vi "AuxSetCurrent.vi"(6 "Enabled?":bool=TRUE, 8 "error in":errorcluster, 9 "VISA resource name":refnum<visa-resource-name>="COM8", 10 "Function select":enum16{"Init", "Set", "Close"}(ring)=enum."Set", 11 "current /mA":dbl) -> (0 "error out":errorcluster, 1 "VISA resource name out":refnum<visa-resource-name>, 3 "output str":string)   [LabVIEW 2019]
uses:
  <vilib>/Instr/_visa.llb/VISA Configure Serial Port (Instr).vi
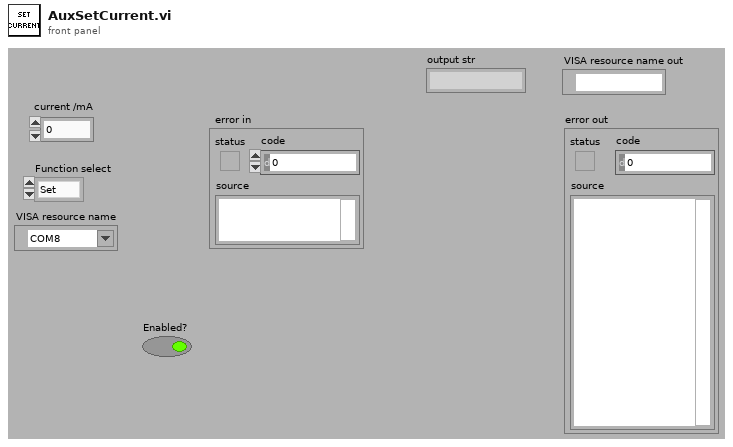
[diagram p1: front panel]
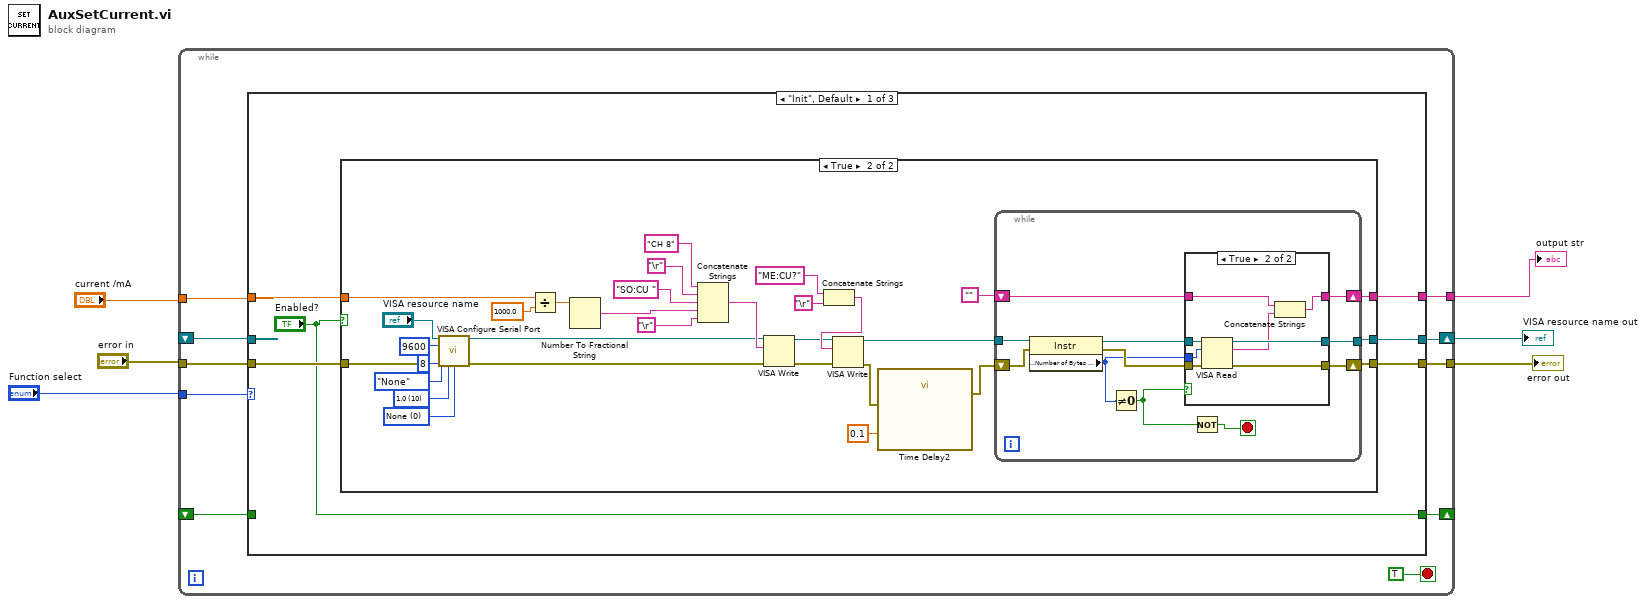
[diagram p0: block diagram]
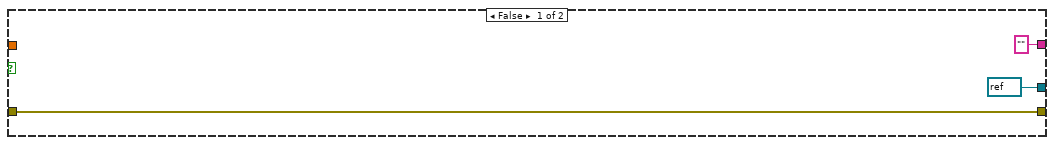
[diagram p2: hidden frame]
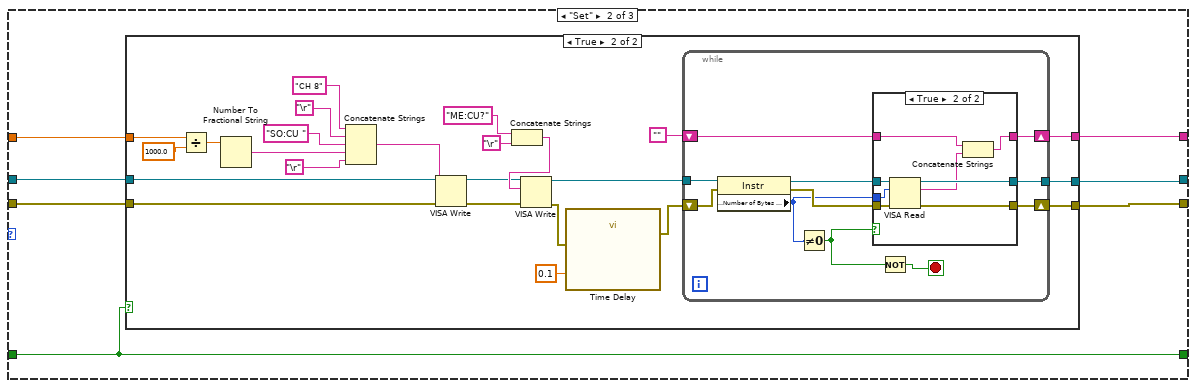
[diagram p4: hidden frame]
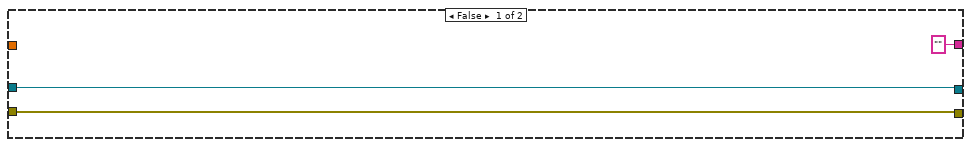
[diagram p5: hidden frame]
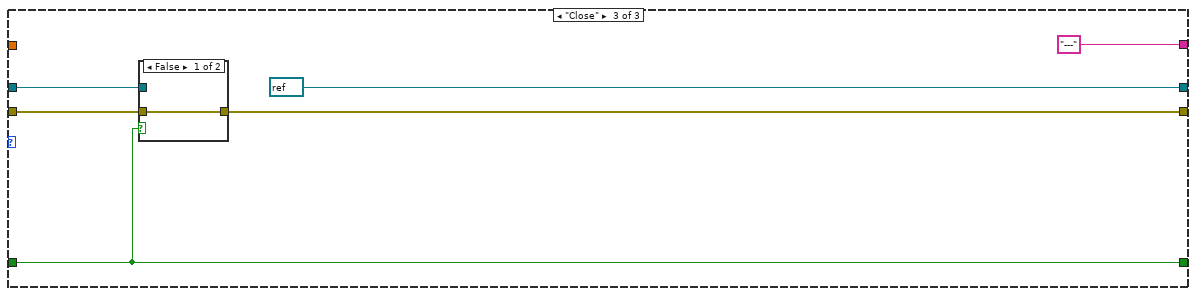
[diagram p7: hidden frame]
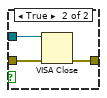
[diagram p8: hidden frame]
diagram:
  n1 = while {
    shift-right: [w15] -> w2
    shift-left: _ -> [w14]
    tunnel: "Function select" -> [w13]
    tunnel: "current /mA" -> [w12]
    tunnel: [w11] -> w4
    tunnel: "error in" -> [w10]
    tunnel: [w9] -> w1
    shift-right: [w8] -> _
    shift-left: _ -> [w7]
    stop <- TRUE stop-if-true
    n2 = case shown="\"Init\", Default" w13 {
      tunnel: [w19 w82 refnum<visa-resource-name> refnum ("VISA resource name out")] -> w15
      tunnel: w14 -> [_ w83 w140]
      tunnel: w12 -> [w21 w85 _]
      tunnel: [w18 w81 w137] -> w11
      tunnel: w10 -> [w22 w84 w138]
      tunnel: [w20 w80 "---"] -> w9
      tunnel: ["Enabled?" w79 w135] -> w8
      tunnel: w7 -> [_ w79 w135]
      frame "Init", Default {
        n3 = case shown="True" "Enabled?" {
          tunnel: w22 -> [w24 w50]
          tunnel: w21 -> [_ w39]
          tunnel: ["" w29] -> w20
          tunnel: [refnum<visa-resource-name> refnum ("VISA resource name out") w28] -> w19
          tunnel: [w24 w27] -> w18
          frame False {
          }
          frame True {
            w56 = u16 0 items=["None", "XON/XOFF", "RTS/CTS", "XON/XOFF & RTS/CTS", "DTR/DSR", "XON/XOFF & DTR/DSR"] ("flow control (0:none)")
            w55 = u16 10 items=["1.0"=10, "1.5"=15, "2.0"=20] ("stop bits (10: 1 bit)")
            n4 = call-poly "VISA Configure Serial Port"("VISA resource name"="VISA resource name", "baud rate (9600)"=u32 9600, "data bits (8)"=u16 8, "parity (0:none)"=enum16{"None", "Odd", "Even", "Mark", "Space"}."None", "error in (no error)"=w50, "stop bits (10: 1 bit)"=w55, "flow control (0:none)"=w56) -> ("VISA resource name out"=w40:refnum<visa-resource-name>, "error out"=w41:errorcluster)  [unwired: 7 in]
            n5 = Divide(x=w39, y=1000.0) -> (x/y=w45:dbl)
            n6 = Number To Fractional String(number=w45) -> (F-format string=w42:string)  [unwired: 3 in]
            n7 = Concatenate Strings("CH 8" ("write buffer"), "\r", "SO:CU ", w42, "\r") -> (w46:string)
            n8 = VISA Write(VISA resource name=w40, write buffer=w46, error in (no error)=w41) -> (VISA resource name out=w31:refnum<visa-resource-name>, error out=w30:errorcluster)  [unwired: 1 out]
            n9 = Concatenate Strings("ME:CU?" ("write buffer"), "\r") -> (w35:string)
            n10 = VISA Write(VISA resource name=w31, write buffer=w35, error in (no error)=w30) -> (VISA resource name out=w36:refnum<visa-resource-name>, error out=w38:errorcluster)  [unwired: 1 out]
            n11 = call "Time Delay2"("error in (no error)"=w38, "Delay Time (s)"=0.1) -> ("error out"=w37:errorcluster)  [unwired: 9 in]
            n12 = while {
              tunnel: w36 -> [w66]
              tunnel: [w63] -> w28
              shift-right: [w62] -> w27
              shift-left: w37 -> [w67]
              shift-right: [w57] -> w29
              shift-left: "" -> [w58]
              stop <- w60 stop-if-true
              n13 = property class="Instr"(reference=w66, error in=w67) -> (reference out=w65:refnum<visa-resource-name>, error out=w64:errorcluster, "Serial Settings:Number of Bytes at Serial Port"=w61:u32)
              n14 = Not Equal To 0?(x=w61) -> (x != 0?=w59:bool)
              n15 = case shown="True" w59 {
                tunnel: w65 -> [w70 w78]
                tunnel: w64 -> [w69 w77]
                tunnel: [w70 w75] -> w63
                tunnel: [w69 w74] -> w62
                tunnel: w61 -> [_ w76]
                tunnel: w58 -> [w68 w73]
                tunnel: [w68 w71] -> w57
                frame False {
                }
                frame True {
                  n16 = VISA Read(VISA resource name=w78, byte count=w76, error in (no error)=w77) -> (VISA resource name out=w75:refnum<visa-resource-name>, read buffer=w72:string, error out=w74:errorcluster)  [unwired: 1 out]
                  n17 = Concatenate Strings(w73, w72) -> (w71:string)
                }
              }
              n18 = Not(x=w59) -> (.not. x?=w60:bool)
            }
          }
        }
      }
      frame "Set" {
        n19 = case shown="True" w79 {
          tunnel: w85 -> [_ w104]
          tunnel: w84 -> [w88 w103]
          tunnel: w83 -> [w87 w102]
          tunnel: [w87 w91] -> w82
          tunnel: [w88 w90] -> w81
          tunnel: ["" w89] -> w80
          frame False {
          }
          frame True {
            n20 = Divide(x=w104, y=1000.0) -> (x/y=w108:dbl)
            n21 = Number To Fractional String(number=w108) -> (F-format string=w105:string)  [unwired: 3 in]
            n22 = Concatenate Strings("CH 8" ("write buffer"), "\r", "SO:CU ", w105, "\r") -> (w109:string)
            n23 = VISA Write(VISA resource name=w102, write buffer=w109, error in (no error)=w103) -> (VISA resource name out=w93:refnum<visa-resource-name>, error out=w92:errorcluster)  [unwired: 1 out]
            n24 = Concatenate Strings("ME:CU?" ("write buffer"), "\r") -> (w98:string)
            n25 = VISA Write(VISA resource name=w93, write buffer=w98, error in (no error)=w92) -> (VISA resource name out=w96:refnum<visa-resource-name>, error out=w94:errorcluster)  [unwired: 1 out]
            n26 = call "Time Delay"("error in (no error)"=w94, "Delay Time (s)"=0.1) -> ("error out"=w95:errorcluster)  [unwired: 9 in]
            n27 = while {
              tunnel: w96 -> [w122]
              tunnel: [w119] -> w91
              shift-right: [w118] -> w90
              shift-left: w95 -> [w123]
              shift-right: [w113] -> w89
              shift-left: "" -> [w114]
              stop <- w116 stop-if-true
              n28 = property class="Instr"(reference=w122, error in=w123) -> (reference out=w121:refnum<visa-resource-name>, error out=w120:errorcluster, "Serial Settings:Number of Bytes at Serial Port"=w117:u32)
              n29 = Not Equal To 0?(x=w117) -> (x != 0?=w115:bool)
              n30 = case shown="True" w115 {
                tunnel: w121 -> [w126 w134]
                tunnel: w120 -> [w125 w133]
                tunnel: [w126 w131] -> w119
                tunnel: [w125 w130] -> w118
                tunnel: w117 -> [_ w132]
                tunnel: w114 -> [w124 w129]
                tunnel: [w124 w127] -> w113
                frame False {
                }
                frame True {
                  n31 = VISA Read(VISA resource name=w134, byte count=w132, error in (no error)=w133) -> (VISA resource name out=w131:refnum<visa-resource-name>, read buffer=w128:string, error out=w130:errorcluster)  [unwired: 1 out]
                  n32 = Concatenate Strings(w129, w128) -> (w127:string)
                }
              }
              n33 = Not(x=w115) -> (.not. x?=w116:bool)
            }
          }
        }
      }
      frame "Close" {
        n34 = case shown="False" w135 {
          tunnel: w140 -> [_ w144]
          tunnel: w138 -> [w141 w143]
          tunnel: [w141 w142] -> w137
          frame False {
          }
          frame True {
            n35 = VISA Close(VISA resource name=w144, error in (no error)=w143) -> (error out=w142:errorcluster)
          }
        }
      }
    }
  }
  "error out" <- w4
  "VISA resource name out" <- w2
  "output str" <- w1
